vi "Update Attributes B.vi"(7 "Attributes in":refnum<class "Attributes.lvclass">, 10 "Actors":refnum<class "Actor.lvclass">[](array[class])) -> (5 "Attributes out":refnum<class "Attributes.lvclass">)   [LabVIEW 2020, in "jettl.lvlib"]
uses:
  jettl.lvlib
  Attributes/Attributes.lvclass
  Actor/Actor.lvclass
  Attributes.ctl
  Transport/Transport.lvclass
  Msgs.ctl
  Msg/Msg.lvclass
  Base Attributes/Base Attributes/Base Attributes.lvclass/Base Attributes.ctl
  Base Attributes/Base Attributes/Base Attributes.lvclass
  C:/git/jettl/src/jettl/jettl/Attributes/Attributes.lvclass
  Base Attributes/Base Attributes.lvlib
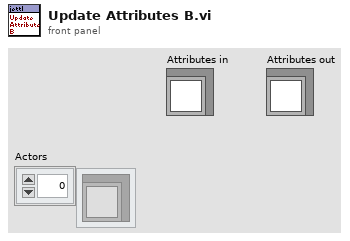
[diagram p1: front panel]
types:
  T1 = typedef "jettl.lvlib/Attributes.ctl" = cluster{"Unified Msgs":T2, "Edge Actors":refnum<class "Actor.lvclass">[], "Core Actors":refnum<class "Actor.lvclass">[], "Parent Attributes":refnum<class "Attributes.lvclass">, "Root":bool, "App Ref":refnum<vi>, "UID":string, "Transport":refnum<class "Transport.lvclass">, "VI Ref":refnum<vi>, "Actors":refnum<class "Actor.lvclass">[]}
  T2 = typedef "jettl.lvlib/Msgs.ctl" = set{refnum<class "Msg.lvclass">}
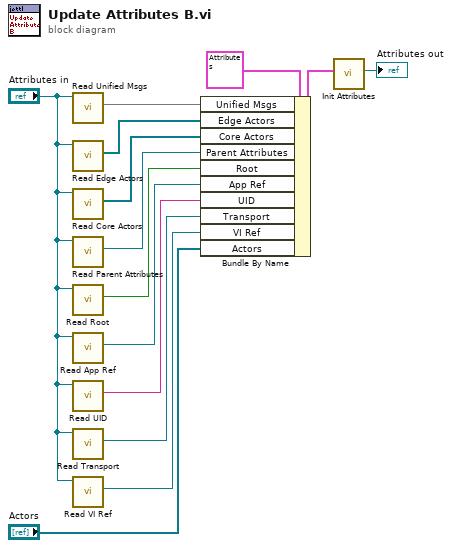
[diagram p0: block diagram]
diagram:
  n1 = call-dynamic "Read Unified Msgs.vi"("Attributes in"="Attributes in") -> ("Unified Msgs"=w3:T2)  [unwired: 10 in]
  n2 = call-dynamic "Read Edge Actors.vi"("Attributes in"="Attributes in") -> ("Edge Actors"=w2:refnum<class "Actor.lvclass">[])  [unwired: 10 in]
  n3 = call-dynamic "Read Core Actors.vi"("Attributes in"="Attributes in") -> ("Core Actors"=w4:refnum<class "Actor.lvclass">[])  [unwired: 10 in]
  n4 = call-dynamic "Read Parent Attributes.vi"("Attributes in"="Attributes in") -> ("Parent Attributes"=w5:refnum<class "Attributes.lvclass">)  [unwired: 10 in]
  n5 = call-dynamic "Read Root.vi"("Attributes in"="Attributes in") -> ("Root"=w6:bool)  [unwired: 10 in]
  n6 = call-dynamic "Read App Ref.vi"("Attributes in"="Attributes in") -> ("App Ref"=w7:refnum<vi>)  [unwired: 10 in]
  n7 = call-dynamic "Read UID.vi"("Attributes in"="Attributes in") -> ("UID"=w8:string)  [unwired: 10 in]
  n8 = call-dynamic "Read Transport.vi"("Attributes in"="Attributes in") -> ("Transport"=w9:refnum<class "Transport.lvclass">)  [unwired: 10 in]
  n9 = call-dynamic "Read VI Ref.vi"("Attributes in"="Attributes in") -> ("VI Ref"=w10:refnum<vi>)  [unwired: 10 in]
  n10 = Bundle By Name(cluster=T1 {"Unified Msgs"={}, "Edge Actors"=[], "Core Actors"=[], "Parent Attributes"=refnum, "Root"=FALSE, "App Ref"=refnum, "UID"="", "Transport"=refnum, "VI Ref"=refnum, "Actors"=[]} ("Attributes"), "Unified Msgs"=w3, "Edge Actors"=w2, "Core Actors"=w4, "Parent Attributes"=w5, "Root"=w6, "App Ref"=w7, "UID"=w8, "Transport"=w9, "VI Ref"=w10, "Actors"="Actors") -> (w12:T1)
  n11 = call "Init Attributes.vi"("Attributes"=w12) -> ("Attributes"=→"Attributes out":refnum<class "Attributes.lvclass">)  [unwired: 10 in]
